vi "GetFreq.vi"(0 "Session In":refnum<visa-resource-name>="TCPIP0::169.254.70.180::inst0::INSTR", 11 "error in":errorcluster {"code" format="%.0x"}, 12 "CHAN(1)":i32=1) -> (2 "NumPoi":dbl, 3 "Freq(ary)":dbl[](array[numeric]), 4 "Session Out":refnum<visa-resource-name>, 15 "error out":errorcluster {"code" format="%.0x"})   [LabVIEW 2018]
doc: "Launches the Instrument I/O Assistant, which you can use to communicate with message-based instruments and graphically parse the response. For example you can communicate with an instrument that uses a serial, Ethernet, or GPIB interface."
panel:
  out "Step":dbl
  out "F_Stop":dbl
  out "F_Start":dbl
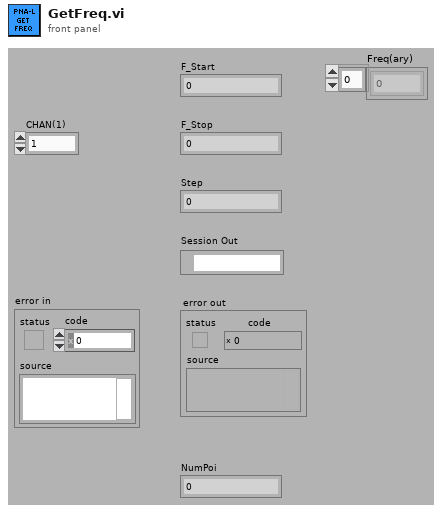
[diagram p1: front panel]
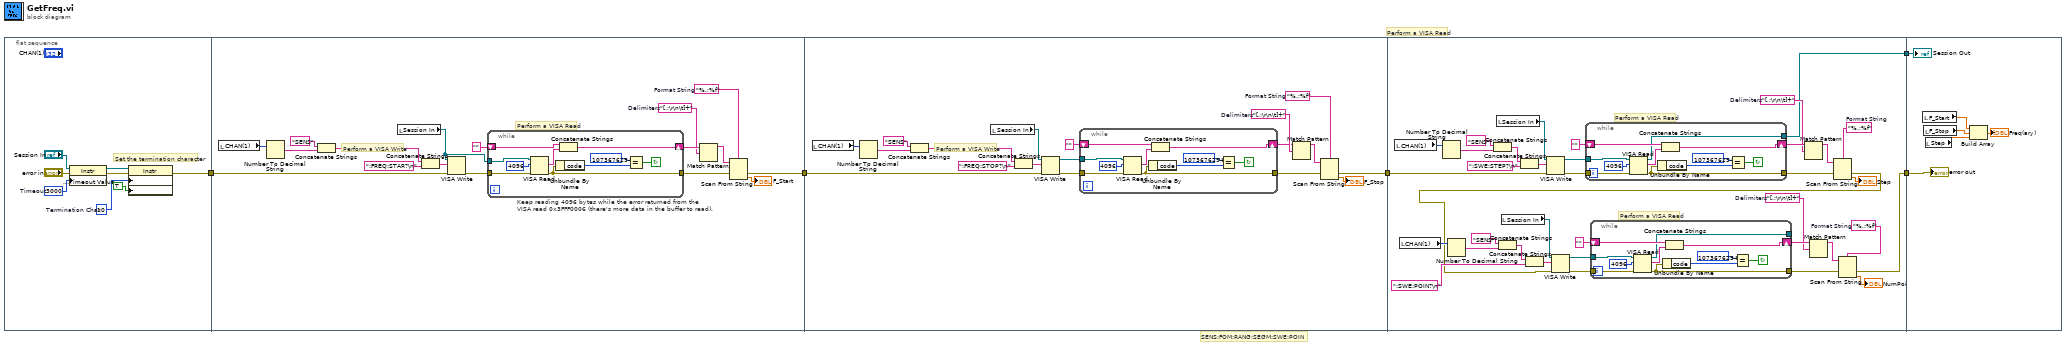
[diagram p0: block diagram]
diagram:
  # "SENS:FOM:RANG:SEGM:SWE:POIN"
  # "Perform a VISA Read"
  n1 = flat-sequence {
    tunnel: [w9] -> w5
    tunnel: w5 -> [w17]
    tunnel: [w14] -> w4
    tunnel: w4 -> [w51]
    tunnel: [w43] -> w3
    tunnel: w3 -> [w87]
    tunnel: [w69] -> w2
    tunnel: [w88] -> w1
    tunnel: w2 -> [w132]
    tunnel: w1 -> [w131]
    frame #0 {
      w8 = u8 10  # Termination Char
      w12 = u32 3000  # Timeout
      # "Set the termination character"
      n2 = property class="Instr"(reference="Session In", error in="error in", "General Settings:Timeout Value"=w12) -> (reference out=w7:refnum<visa-resource-name>, error out=w10:errorcluster)
      n3 = property class="Instr"(reference=w7, error in=w10, "Message Based Settings:Termination Character"=w8, "Message Based Settings:Termination Character Enable"=TRUE ("enable")) -> (error out=w9:errorcluster)  [unwired: 1 in]
    }
    frame #1 {
      w21 = "[,;\r\n\t]+"  # Delimiters
      w20 = "%.;%f"  # Format String
      # "Perform a VISA Read"
      # "Keep reading 4096 bytes while the error returned from the\nVISA read 0x3FFF0006 (there's more data in the buffer to read)."
      # "Perform a VISA Write"
      n4 = local read "CHAN(1)"() -> (w29:i32)
      n5 = Number To Decimal String(number=w29) -> (decimal integer string=w22:string)  [unwired: 1 out]
      n6 = Concatenate Strings("SENS" ("staticText"), w22) -> (w25:string)
      n7 = local read "Session In"() -> (w15:refnum<visa-resource-name>)
      n8 = Concatenate Strings(w25, ":FREQ:STAR?\n" ("StaticText")) -> (w24:string)
      n9 = VISA Write(VISA resource name=w15, write buffer=w24, error in (no error)=w17) -> (error out=w23:errorcluster)  [unwired: 2 out]
      n10 = while {
        tunnel: w15 -> [w31]
        shift-left: "" -> [w34]
        shift-right: [w33] -> w27
        tunnel: w23 -> [w32]
        tunnel: [w36] -> w26
        stop <- w38 continue-if-true
        n11 = VISA Read(VISA resource name=w31, byte count=u32 4096 ("byte count (0)"), error in (no error)=w32) -> (read buffer=w35:string, error out=w36:errorcluster)  [unwired: 2 out]
        n12 = Unbundle By Name(w36) -> ("code"=w39:i32)
        n13 = Concatenate Strings(w34, w35) -> (w33:string)
        n14 = Equal?(x=1073676294, y=w39) -> (x = y?=w38:bool)
      }
      n15 = Match Pattern(string=w27, regular expression=w21) -> (before substring=w28:string)  [unwired: 1 in, 3 out]
      n16 = Scan From String(format string=w20, input string=w28, error in=w26) -> (error out=w14:errorcluster, output 1=→"F_Start":dbl)  [unwired: 2 in, 2 out]
    }
    frame #2 {
      w46 = "%.;%f"  # Format String
      w47 = "[,;\r\n\t]+"  # Delimiters
      # "Perform a VISA Write"
      n17 = local read "CHAN(1)"() -> (w58:i32)
      n18 = Number To Decimal String(number=w58) -> (decimal integer string=w56:string)  [unwired: 1 out]
      n19 = Concatenate Strings("SENS" ("staticText"), w56) -> (w57:string)
      n20 = local read "Session In"() -> (w52:refnum<visa-resource-name>)
      n21 = Concatenate Strings(w57, ":FREQ:STOP?\n" ("StaticText")) -> (w53:string)
      n22 = VISA Write(VISA resource name=w52, write buffer=w53, error in (no error)=w51) -> (VISA resource name out=w48:refnum<visa-resource-name>, error out=w50:errorcluster)  [unwired: 1 out]
      n23 = while {
        tunnel: w48 -> [w59]
        shift-left: "" -> [w62]
        shift-right: [w61] -> w45
        tunnel: w50 -> [w60]
        tunnel: [w64] -> w41
        stop <- w66 continue-if-true
        n24 = VISA Read(VISA resource name=w59, byte count=u32 4096 ("byte count (0)"), error in (no error)=w60) -> (read buffer=w63:string, error out=w64:errorcluster)  [unwired: 2 out]
        n25 = Unbundle By Name(w64) -> ("code"=w67:i32)
        n26 = Concatenate Strings(w62, w63) -> (w61:string)
        n27 = Equal?(x=1073676294, y=w67) -> (x = y?=w66:bool)
      }
      n28 = Match Pattern(string=w45, regular expression=w47) -> (before substring=w44:string)  [unwired: 1 in, 3 out]
      n29 = Scan From String(format string=w46, input string=w44, error in=w41) -> (error out=w43:errorcluster, output 1=→"F_Stop":dbl)  [unwired: 2 in, 2 out]
    }
    frame #3 {
      w75 = "[,;\r\n\t]+"  # Delimiters
      w74 = "%.;%f"  # Format String
      w95 = "[,;\r\n\t]+"  # Delimiters
      w94 = "%.;%f"  # Format String
      # "Perform a VISA Read"
      # "Perform a VISA Read"
      n30 = local read "CHAN(1)"() -> (w104:i32)
      n31 = local read "CHAN(1)"() -> (w86:i32)
      n32 = Number To Decimal String(number=w104) -> (decimal integer string=w96:string)  [unwired: 1 out]
      n33 = Number To Decimal String(number=w86) -> (decimal integer string=w78:string)  [unwired: 1 out]
      n34 = Concatenate Strings("SENS" ("staticText"), w96) -> (w99:string)
      n35 = local read "Session In"() -> (w90:refnum<visa-resource-name>)
      n36 = Concatenate Strings("SENS" ("staticText"), w78) -> (w81:string)
      n37 = local read "Session In"() -> (w77:refnum<visa-resource-name>)
      n38 = Concatenate Strings(w99, ":SWE:STEP?\n" ("StaticText")) -> (w98:string)
      n39 = Concatenate Strings(w81, ":SWE:POIN?\n" ("StaticText")) -> (w80:string)
      n40 = VISA Write(VISA resource name=w90, write buffer=w98, error in (no error)=w87) -> (VISA resource name out=w89:refnum<visa-resource-name>, error out=w97:errorcluster)  [unwired: 1 out]
      n41 = while {
        shift-left: "" -> [w120]
        shift-right: [w119] -> w101
        tunnel: w97 -> [w118]
        tunnel: [w122] -> w100
        tunnel: w89 -> [w117]
        tunnel: [w116] -> w88
        stop <- w124 continue-if-true
        n42 = VISA Read(VISA resource name=w117, byte count=u32 4096 ("byte count (0)"), error in (no error)=w118) -> (VISA resource name out=w116:refnum<visa-resource-name>, read buffer=w121:string, error out=w122:errorcluster)  [unwired: 1 out]
        n43 = Unbundle By Name(w122) -> ("code"=w125:i32)
        n44 = Concatenate Strings(w120, w121) -> (w119:string)
        n45 = Equal?(x=1073676294, y=w125) -> (x = y?=w124:bool)
      }
      n46 = Match Pattern(string=w101, regular expression=w95) -> (before substring=w102:string)  [unwired: 1 in, 3 out]
      n47 = Scan From String(format string=w94, input string=w102, error in=w100) -> (error out=w70:errorcluster, output 1=→"Step":dbl)  [unwired: 2 in, 2 out]
      n48 = VISA Write(VISA resource name=w77, write buffer=w80, error in (no error)=w70) -> (VISA resource name out=w76:refnum<visa-resource-name>, error out=w79:errorcluster)  [unwired: 1 out]
      n49 = while {
        shift-left: "" -> [w109]
        shift-right: [w108] -> w83
        tunnel: w79 -> [w107]
        tunnel: [w111] -> w82
        tunnel: w76 -> [w106]
        tunnel: [w105] -> _
        stop <- w113 continue-if-true
        n50 = VISA Read(VISA resource name=w106, byte count=u32 4096 ("byte count (0)"), error in (no error)=w107) -> (VISA resource name out=w105:refnum<visa-resource-name>, read buffer=w110:string, error out=w111:errorcluster)  [unwired: 1 out]
        n51 = Unbundle By Name(w111) -> ("code"=w114:i32)
        n52 = Concatenate Strings(w109, w110) -> (w108:string)
        n53 = Equal?(x=1073676294, y=w114) -> (x = y?=w113:bool)
      }
      n54 = Match Pattern(string=w83, regular expression=w75) -> (before substring=w84:string)  [unwired: 1 in, 3 out]
      n55 = Scan From String(format string=w74, input string=w84, error in=w82) -> (error out=w69:errorcluster, output 1=→"NumPoi":dbl)  [unwired: 2 in, 2 out]
    }
    frame #4 {
      n56 = local read "F_Start"() -> (w129:dbl)
      n57 = local read "F_Stop"() -> (w128:dbl)
      n58 = local read "Step"() -> (w130:dbl)
      n59 = Build Array(w129, w128, w130) -> (→"Freq(ary)":dbl[])
      "error out" <- w132
      "Session Out" <- w131
    }
  }
